vi "formatUnits.vi"(10 "Units":T1[](array[typedef]), 11 "StringFormatter":refnum<class "StringFormatter.lvclass">) -> (2 "Units String":string)   [LabVIEW 2013, in "OpenStringFormatter.lvlib" / "StringFormatter.lvclass"]
uses:
  StringFormatter.lvclass
  <vilib>/Utility/VariantDataType/UnitInfo.ctl
  <vilib>/Utility/VariantDataType/UnitType.ctl
  <vilib>/Utility/VariantDataType/VariantType.lvlib
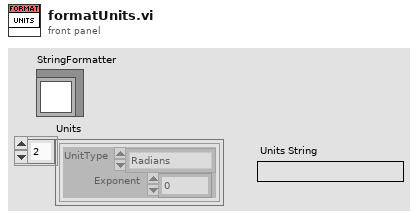
[diagram p1: front panel]
types:
  T1 = typedef "VariantType.lvlib/UnitInfo.ctl" = cluster{"UnitType":T2, "Exponent":i16}
  T2 = typedef "VariantType.lvlib/UnitType.ctl" = enum16{"Radians", "Steradians", "Seconds", "Meters", "Kilograms", "Amperes", "Kelvins", "Moles", "Candelas", "InvalidUnit"}
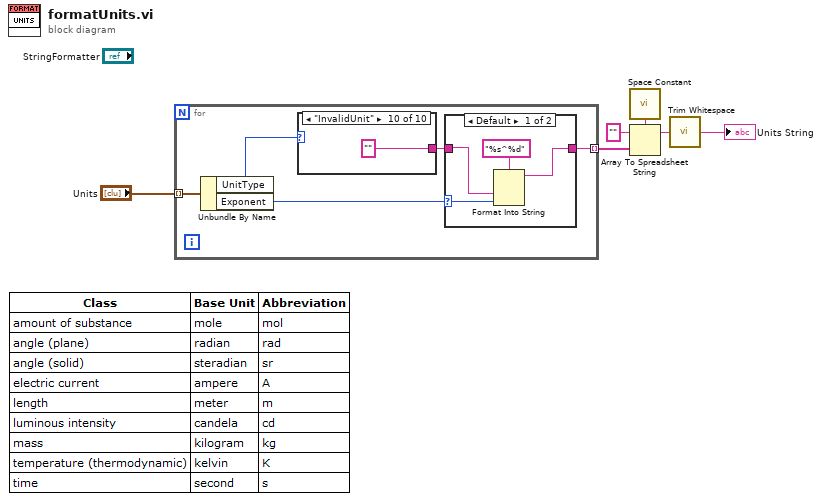
[diagram p0: block diagram]
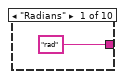
[diagram p3: hidden frame]
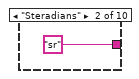
[diagram p4: hidden frame]
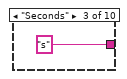
[diagram p5: hidden frame]
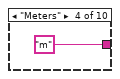
[diagram p6: hidden frame]
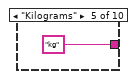
[diagram p7: hidden frame]
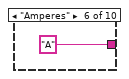
[diagram p8: hidden frame]
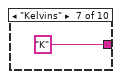
[diagram p9: hidden frame]
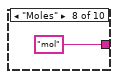
[diagram p10: hidden frame]
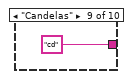
[diagram p11: hidden frame]
diagram:
  n1 = for {
    tunnel: "Units" -> [w11] mode=indexing
    tunnel: [w8] -> w4 mode=indexing
    n2 = Unbundle By Name(w11) -> ("UnitType"=w10:T2, "Exponent"=w9:i16)
    n3 = case shown="\"InvalidUnit\"" w10 {
      tunnel: ["rad" "sr" "s" "m" "kg" "A" "K" "mol" "cd" ""] -> w7
      frame "Radians" {
      }
      frame "Steradians" {
      }
      frame "Seconds" {
      }
      frame "Meters" {
      }
      frame "Kilograms" {
      }
      frame "Amperes" {
      }
      frame "Kelvins" {
      }
      frame "Moles" {
      }
      frame "Candelas" {
      }
      frame "InvalidUnit" {
      }
    }
    n4 = case shown="Default" w9 {
      selector: w9 -> [w15 _]
      tunnel: [w13 w16] -> w8
      tunnel: w7 -> [w14 w16]
      frame Default {
        n5 = Format Into String(format string="%s^%d", w14, w15) -> (resulting string=w13:string)  [unwired: 2 in, 1 out]
      }
      frame 1 {
      }
    }
  }
  n6 = call <vilib>:"Space Constant.vi"() -> ("String"=w3:string)
  n7 = Array To Spreadsheet String(delimiter (Tab)=w3, array=w4, 3:"" ("format string")) -> (spreadsheet string=w5:string)
  n8 = call <vilib>:"Trim Whitespace.vi"("string"=w5) -> ("trimmed string"=→"Units String":string)  [unwired: 1 in]
